vi "Initialize Hardware.vi"(8 "error in (no error)":errorcluster, 9 "DAQ Type":enum16{"Hardware", "Simulation"}(ring), 10 "Serial Parameter":T1={"VISA resource name"="", "baud rate (9600)"=9600, "data bits (8)"=8, "parity (0:none)"=enum."None", "stop bits (10: 1 bit)"=10, "flow control (0:none)"=0, "termination char\n(0xA = '\\n' = LF) "=10, "Enable Termination\nChar (T)"=TRUE, "timeout (10sec)"=10000} {"flow control (0:none)" items=["None", "XON/XOFF", "RTS/CTS", "XON/XOFF & RTS/CTS", "DTR/DSR", "XON/XOFF & DTR/DSR"]; "stop bits (10: 1 bit)" items=["None", "Odd", "Even", "Mark", "Space"]; "termination char\n(0xA = '\\n' = LF)" format="%.0x"}, 11 "Serial Device in":refnum<class "Serial Device.lvclass">) -> (0 "error out":errorcluster, 3 "Serial Device out":refnum<class "Serial Device.lvclass">)   [LabVIEW 2021, in "Serial Hardware.lvlib" / "Serial Device.lvclass"]
uses:
  Serial Device.lvclass
  Serial Parameter.ctl
  Serial Device.lvclass/Serial Device.ctl
  <vilib>/Instr/_visa.llb/VISA Configure Serial Port (Instr).vi
  Serial Hardware.lvlib
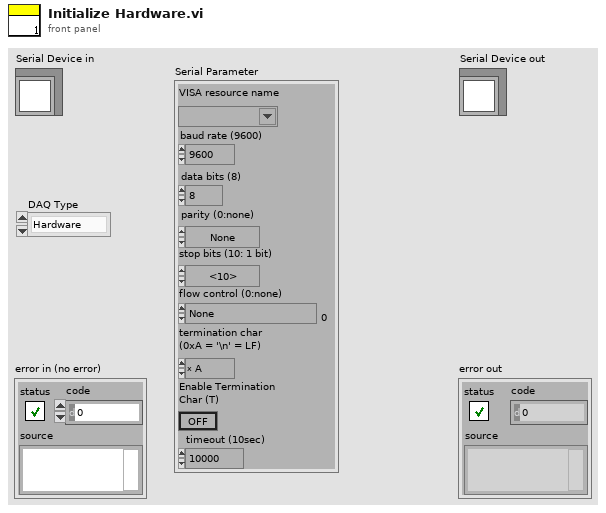
[diagram p1: front panel]
types:
  T1 = typedef "Serial Hardware.lvlib/Serial Parameter.ctl" = cluster{"VISA resource name":refnum<visa-resource-name>, "baud rate (9600)":u32, "data bits (8)":u16, "parity (0:none)":enum16{"None", "Odd", "Even", "Mark", "Space"}, "stop bits (10: 1 bit)":u16, "flow control (0:none)":u16, "termination char\n(0xA = '\\n' = LF) ":u8, "Enable Termination\nChar (T)":bool, "timeout (10sec)":u32}
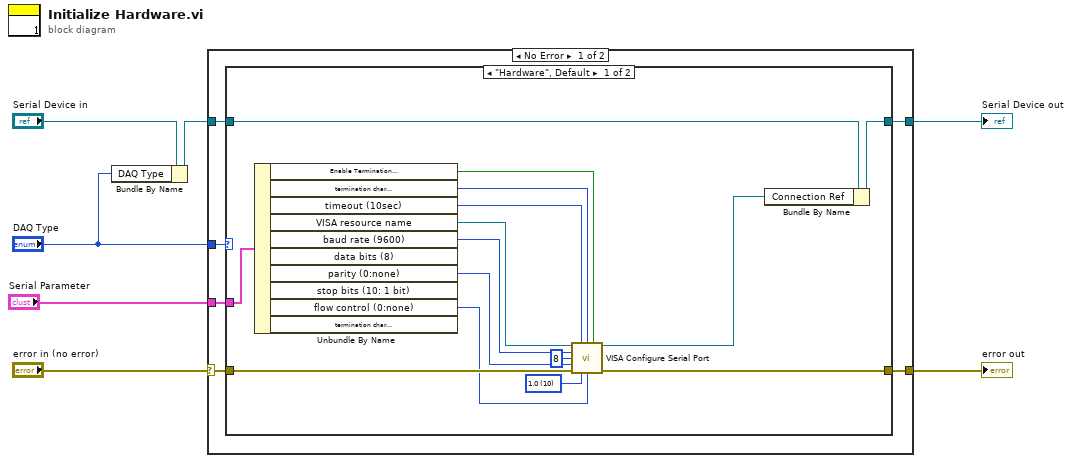
[diagram p0: block diagram]
diagram:
  n1 = Bundle By Name(cluster="Serial Device in", "DAQ Type"="DAQ Type") -> (w5:refnum<class "Serial Device.lvclass">)
  n2 = case shown="No Error" "error in (no error)" {
    selector: "error in (no error)" -> [w10 w31]
    tunnel: w5 -> [w13 w32]
    tunnel: "DAQ Type" -> [w12 _]
    tunnel: [w11 w32] -> w3
    tunnel: [w8 w31] -> w2
    tunnel: "Serial Parameter" -> [w9 _]
    frame No Error {
      n3 = case shown="\"Hardware\", Default" w12 {
        tunnel: w13 -> [w28 w29]
        tunnel: [w17 w29] -> w11
        tunnel: w10 -> [w26 w30]
        tunnel: w9 -> [w27 _]
        tunnel: [w25 w30] -> w8
        frame "Hardware", Default {
          w15 = u16 10 items=["1.0"=10, "1.5"=15, "2.0"=20] ("stop bits (10: 1 bit)")
          n4 = Unbundle By Name(w27) -> ("Enable Termination\nChar (T)"=w18:bool, "termination char\n(0xA = '\\n' = LF)"=w19:u8, "timeout (10sec)"=w20:u32, "VISA resource name"=w24:refnum<visa-resource-name>, "baud rate (9600)"=w23:u32, "parity (0:none)"=w22:enum16{"None", "Odd", "Even", "Mark", "Space"}, "flow control (0:none)"=w21:u16)  [unwired: 3 out]
          n5 = call-poly "VISA Configure Serial Port"("VISA resource name"=w24, "timeout (10sec)"=w20, "termination char\n(0xA = '\\n' = LF)"=w19, "Enable Termination\nChar (T)"=w18, "baud rate (9600)"=w23, "data bits (8)"=u16 8, "parity (0:none)"=w22, "error in (no error)"=w26, "stop bits (10: 1 bit)"=w15, "flow control (0:none)"=w21) -> ("VISA resource name out"=w16:refnum<visa-resource-name>, "error out"=w25:errorcluster)  [unwired: 4 in]
          n6 = Bundle By Name(cluster=w28, "Connection Ref"=w16) -> (w17:refnum<class "Serial Device.lvclass">)
        }
        frame "Simulation" {
        }
      }
    }
    frame Error {
    }
  }
  "error out" <- w2
  "Serial Device out" <- w3
